vi "Prepare.vi"(6 "notifier in":refnum<notifier>, 8 "error in":errorcluster, 10 "Iterator Settings":T1={"Prepare timeout (ms)"=200, "Iterate timeout (ms)"=50, "Conclude timeout (ms)"=200, "Iterate period (ms)"=200, "Number of iterations"=5, "Stop Condition"=enum."None", "Time before stop (ms)"=5, "Prepare Msg"=refnum, "Iterate Msg"=refnum, "Conclude Msg"=refnum, "Error Handler"=refnum}, 11 "Caller Enqueuer in":refnum<class "Message Enqueuer.lvclass">) -> (0 "error out":errorcluster, 2 "Reply":bool, 3 "Caller Enqueuer out":refnum<class "Message Enqueuer.lvclass">)   [LabVIEW 2016, in "Iterator Actor.lvlib" / "Iterator Actor.lvclass"]
doc: "Calls the Prepare method of the Client and receives its responce."
uses:
  Iterator Actor.lvclass
  Iterator Settings.ctl
  Iterator Actor Abstract Messages/Iterator Reply Msg/Iterator Reply Msg.lvclass
  C:/Program Files (x86)/National Instruments/LabVIEW 2016/vi.lib/ActorFramework/Message/Message.lvclass
  Iterator Actor Abstract Messages/Iterator Report Error Msg/Iterator Report Error Msg.lvclass
  Stop Condition.ctl
  <vilib>/ActorFramework/Message Enqueuer/Message Enqueuer.lvclass
  Iterator Actor Abstract Messages/Iterator Reply Msg/Iterator Reply Msg.lvclass/Iterator Reply Msg.ctl
  <vilib>/ActorFramework/Message Enqueuer/Message Enqueuer.lvclass/Message Enqueuer.ctl
  Iterator Errors.ctl
  <vilib>/ActorFramework/Message Enqueuer/Enqueue.vi
  <vilib>/ActorFramework/Message Priority Queue/Priority Enqueue.vi
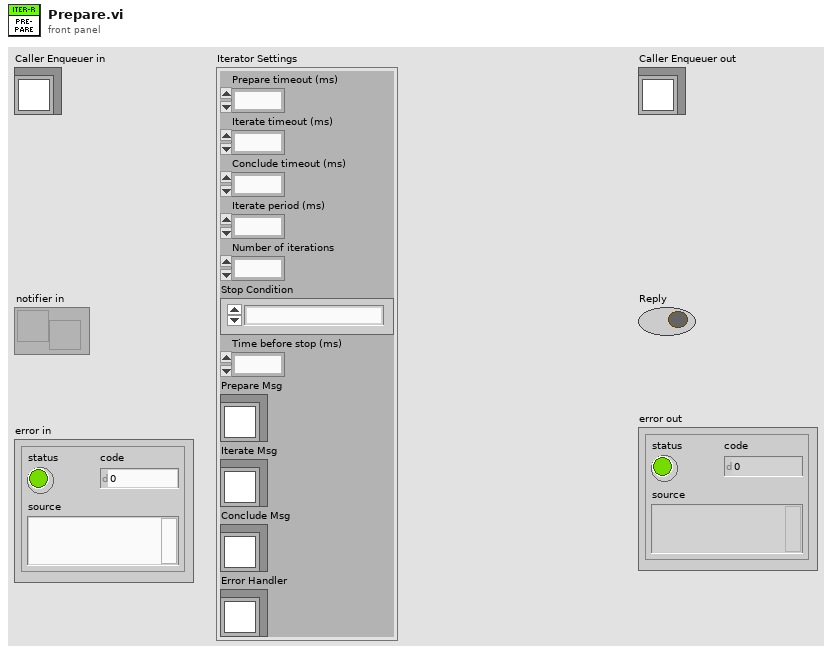
[diagram p1: front panel]
types:
  T1 = typedef "Iterator Actor.lvlib/Iterator Actor.lvclass/Iterator Settings.ctl" = cluster{"Prepare timeout (ms)":i32, "Iterate timeout (ms)":i32, "Conclude timeout (ms)":i32, "Iterate period (ms)":i32, "Number of iterations":i32, "Stop Condition":T2, "Time before stop (ms)":i32, "Prepare Msg":refnum<class "Iterator Reply Msg.lvclass">, "Iterate Msg":refnum<class "Iterator Reply Msg.lvclass">, "Conclude Msg":refnum<class "Iterator Reply Msg.lvclass">, "Error Handler":refnum<class "Iterator Report Error Msg.lvclass">}
  T2 = typedef "Iterator Actor.lvlib/Iterator Actor.lvclass/Stop Condition.ctl" = enum16{"None", "Number of iterations", "Time elapsed", "Iteration result"}
  T3 = typedef "Iterator Actor.lvlib/Iterator Actor.lvclass/Iterator Errors.ctl" = enum16{"Input parameters are not valid", "Preparation call timed out", "Iteration call timed out", "Conclusion call timed out"}
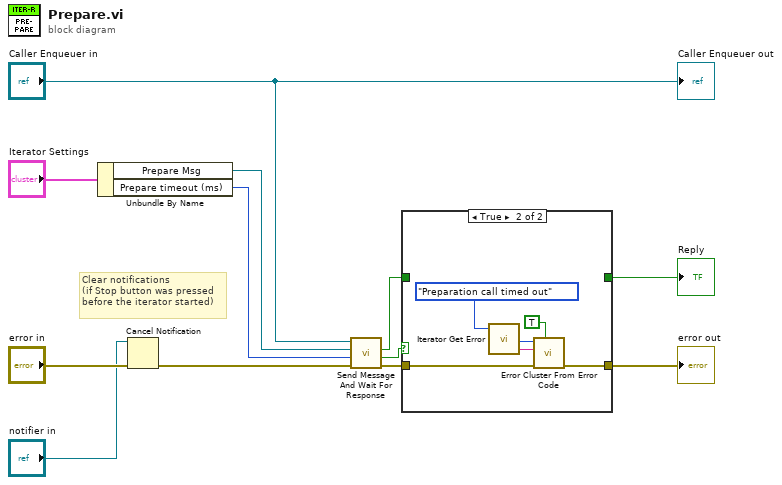
[diagram p0: block diagram]
diagram:
  # "Clear notifications\n(if Stop button was pressed\nbefore the iterator started)"
  n1 = Unbundle By Name("Iterator Settings") -> ("Prepare Msg"=w11:refnum<class "Iterator Reply Msg.lvclass">, "Prepare timeout (ms)"=w12:i32)
  n2 = Cancel Notification(0:"notifier in", 3:"error in") -> (11:w2:errorcluster)  [unwired: 2 out]
  n3 = call "Send Message And Wait For Response.vi"("error in (no error)"=w2, "timeout in ms (-1)"=w12, "Original Message"=w11, "Message Enqueuer in"="Caller Enqueuer in") -> ("error out"=w5:errorcluster, "timed out?"=w7:bool, "Reply"=w8:bool)  [unwired: 4 in, 1 out]
  n4 = case shown="True" w7 {
    tunnel: w5 -> [w13 w17]
    tunnel: [w13 w16] -> w6
    tunnel: w8 -> [w14 _]
    tunnel: [w14 _] -> w9
    frame False {
    }
    frame True {
      n5 = call "Iterator Get Error.vi"("Error"=Iterator_Errors."Preparation call timed out") -> ("source"=w19:string, "code"=w18:i32)  [unwired: 2 in, 1 out]
      n6 = call <vilib>:"Error Cluster From Error Code.vi"("show call chain? (False)"=TRUE ("is warning? (False)"), "error in (no error)"=w17, "error message (\"\")"=w19, "error code (0)"=w18) -> ("error out"=w16:errorcluster)  [unwired: 5 in]
    }
  }
  "Reply" <- w9
  "error out" <- w6
  "Caller Enqueuer out" <- "Caller Enqueuer in"
